vi "7-JUNKOLDOCU.vi"() -> ()   [LabVIEW 2010]
uses:
  7-OCU/7.0-Global.vi
  7-OCU/TabEnum.ctl
  6-OCU Neurons/6.1-UDP Saitek.ctl
  6-OCU Neurons/MDF LatLong.ctl
  6-OCU Neurons/6.1-Act.ctl
  <vilib>/Utility/inputDevices.llb/joystickAcquire.vi
panel:
  in  "Stop Loops 2":bool
  out "Ogrid":u8[][](graph)
  out "MDF Array Out":T1[](array[typedef]) {"Latitude (waypoint)" format="%#_8g"; "Longitude  (waypoint)" format="%#_8g"}
  out "PlanMission":bool
  out "initialized MDF":T1[](array[typedef]) {"Latitude (waypoint)" format="%#_8g"; "Longitude  (waypoint)" format="%#_8g"}
  out "Process loop":bool
  out "AutoMode":bool
  out "ManualMode":bool
  in  "Stop Loops":bool
  out "Startup&Shutdown":bool
  out "Main Tab":string
  in  "Main Tab Interface":T2
  out "Drive Motor Check":bool
  out "Steer Motor Check":bool
  out "LIDAR Motor Check":bool
  out "Vector Nav Check":bool
  in  "Path":path=path "C:/Users/jmccandless/Documents/Olin/S6 - S11/Robotics/Dave Brain 5/Graphics/PNG/olin_o.png"
  out "ignore me 2":bool
  out "ignore me":bool
  out "Way Point Index":i32
  out "Draw??":bool
  in  "Pen Color":u32(colorbox)=15671808
  in  "Select Pen Attributes":T3={"Width"=1, "Style"=enum."Solid"}
  out "Current Waypoint":T1={"Waypoint #"=2.0, "Latitude (waypoint)"=0.0, "Longitude  (waypoint)"=0.0, "Vel (desired)"=0.0, "Dwell Time"=0.0, "Behavior"=enum."OpenFieldTransit", "Expand1"=0.0, "Expand2"=0.0, "Expand3"=0.0} {"Latitude (waypoint)" format="%#_8g"; "Longitude  (waypoint)" format="%#_8g"}
  in  "RobotSpeed_Leg":dbl(slide) min=0.0 max=4.0 step=0.01 scale=0.0..4.0
  in  "Select Your Behavior":T4(ring)
  in  "Exit Planning":bool
  in  "Load From File":bool
  in  "Save to File":bool
  out "MissionDefFile":picture
  out "Saitek Controler 2":T5 {"Right" scale=-32767.0..32767.0; "Left" scale=-32767.0..32767.0; "Yaw" scale=-32767.0..32767.0; "Roll" scale=-32767.0..32767.0; "Pitch" scale=-32767.0..32767.0}
  out "7.7.1 ManualMode Main Controls":T6 {"6.1-Saitek Controller"."Right" scale=-32767.0..32767.0; "6.1-Saitek Controller"."Left" scale=-32767.0..32767.0; "6.1-Saitek Controller"."Yaw" scale=-32767.0..32767.0; "6.1-Saitek Controller"."Roll" scale=-32767.0..32767.0; "6.1-Saitek Controller"."Pitch" scale=-32767.0..32767.0}
  out "Speed":dbl(knob) scale=0.0..10.0
  out "Heading":dbl(knob) scale=-180.0..180.0
  out "Battery":dbl(slide) scale=0.0..24.0
  out "Time":dbl
  in  "Start Mission":bool
  out "AutoMode Dashboard":T7 {"Battery" scale=0.0..24.0; "Heading" scale=-180.0..180.0; "Speed" scale=0.0..10.0}
  out "7.7.1 AutoMode Main Controls":T6 {"6.1-Saitek Controller"."Right" scale=-32767.0..32767.0; "6.1-Saitek Controller"."Left" scale=-32767.0..32767.0; "6.1-Saitek Controller"."Yaw" scale=-32767.0..32767.0; "6.1-Saitek Controller"."Roll" scale=-32767.0..32767.0; "6.1-Saitek Controller"."Pitch" scale=-32767.0..32767.0}
  out "direction info 2":T8
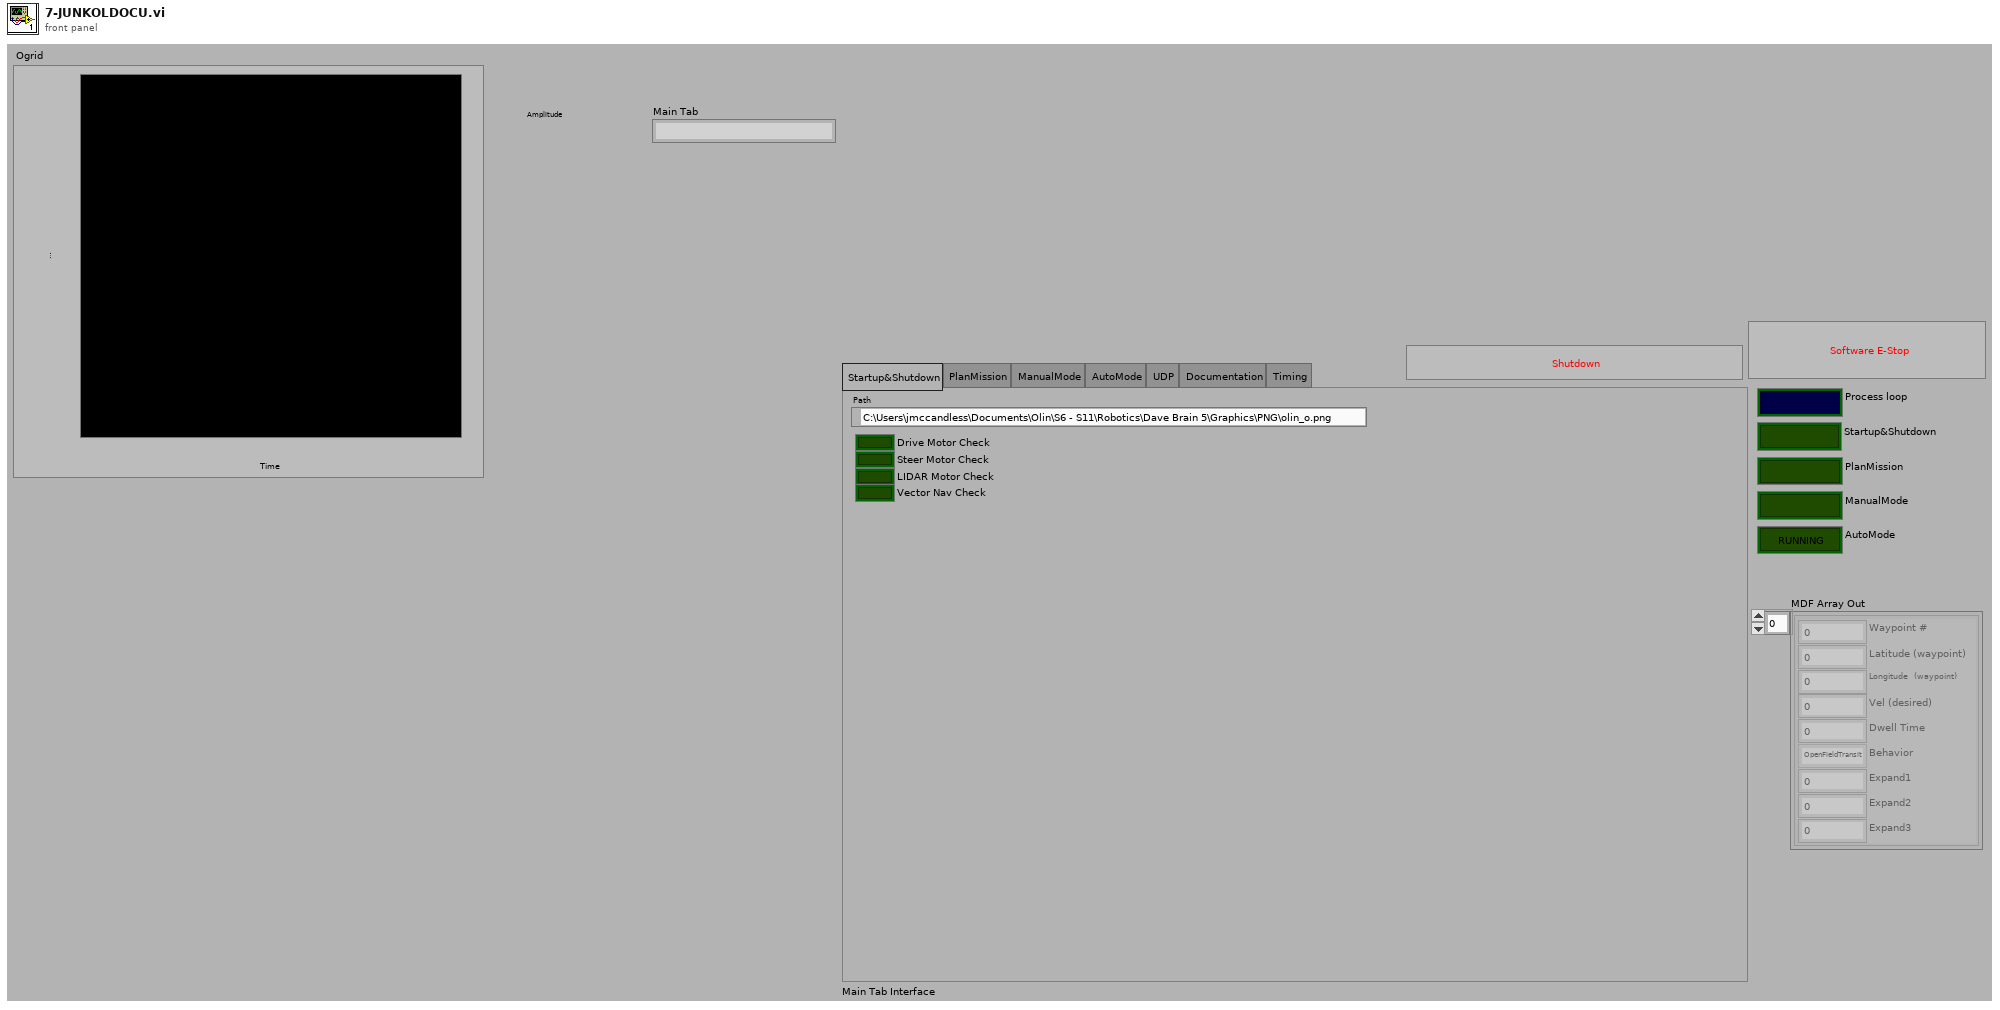
[diagram p1: front panel]
types:
  T1 = typedef "MDF LatLong.ctl" = cluster{"Waypoint #":dbl, "Latitude (waypoint)":ext, "Longitude  (waypoint)":ext, "Vel (desired)":dbl, "Dwell Time":dbl, "Behavior":enum16{"OpenFieldTransit", "WallFollow", "LaneFollow", "ManualMode"}, "Expand1":dbl, "Expand2":dbl, "Expand3":dbl}
  T2 = typedef "TabEnum.ctl" = enum32{"Startup&Shutdown", "PlanMission", "ManualMode", "AutoMode", "UDP", "Documentation", "Timing"}
  T3 = cluster{"Width":u16, "Style":enum32{"Solid", "Dash", "Dot", "DashDot", "DashDotDot"}}
  T4 = enum16{"OpenFieldTransit", "WallFollow", "LaneFollow", "ManualMode"}
  T5 = typedef "6.1-UDP Saitek.ctl" = cluster{"Trig":bool, "2":bool, "3":bool, "4":bool, "5":bool, "6":bool, "7":bool, "8":bool, "9":bool, "10":bool, "11":bool, "Pitch":i32, "Ang":bool[], "Wheel":dbl, "Roll":i32, "Yaw":i32, "Left":i32, "Right":i32}
  T6 = typedef "6.1-Act.ctl" = cluster{"6.1-Saitek Controller":T5, "Joystick Mode":bool, "Shutdown":bool, "Reset":bool, "Begin":bool}
  T7 = cluster{"Speed":dbl, "Heading":dbl, "Battery":dbl, "Time":dbl}
  T8 = cluster{"pov 1":i32, "pov 2":i32, "pov 3":i32, "pov 4":i32}
  T9 = typedef "imagedata.ctl" = cluster{"image type":i32, "image depth":i32, "image":u8[], "mask":u8[], "colors":u32[], "Rectangle":cluster{"left":i16, "top":i16, "right":i16, "bottom":i16}}
  T10 = enum32{"7.1-Act", "7.2-Where", "7.3-What", "7.4-How", "Startup&Shutdown", "PlanMission", "ManualMode", "AutoMode", "UDP", "Documentation", "7.8-Timing"}
  T11 = typedef "LVMouseTypeDef.ctl" = cluster{"Mouse Position":cluster{"X":i32, "Y":i32}, "Mouse Modifiers":cluster{"Button Down":bool, "Shift Mod":bool, "Menu Mod":bool, "Option Mod":bool}}
  T12 = typedef "MDF Array LatLong.ctl" = T1[]
  T13 = cluster{"X axis":i32, "Y axis":i32, "Z axis":i32, "X axis rotation":i32, "Y axis rotation":i32, "Z axis rotation":i32, "U axis":i32, "V axis":i32}
  T14 = cluster{"button 1":bool, "button 2":bool, "button 3":bool, "button 4":bool, "button 5":bool, "button 6":bool, "button 7":bool, "button 8":bool, "button 9":bool, "button 10":bool, "button 11":bool, "button 12":bool, "button 13":bool, "button 14":bool, "button 15":bool, "button 16":bool, "button 17":bool, "button 18":bool, "button 19":bool, "button 20":bool, "button 21":bool, "button 22":bool, "button 23":bool, "button 24":bool, "button 25":bool, "button 26":bool, "button 27":bool, "button 28":bool, "button 29":bool, "button 30":bool, "button 31":bool, "button 32":bool}
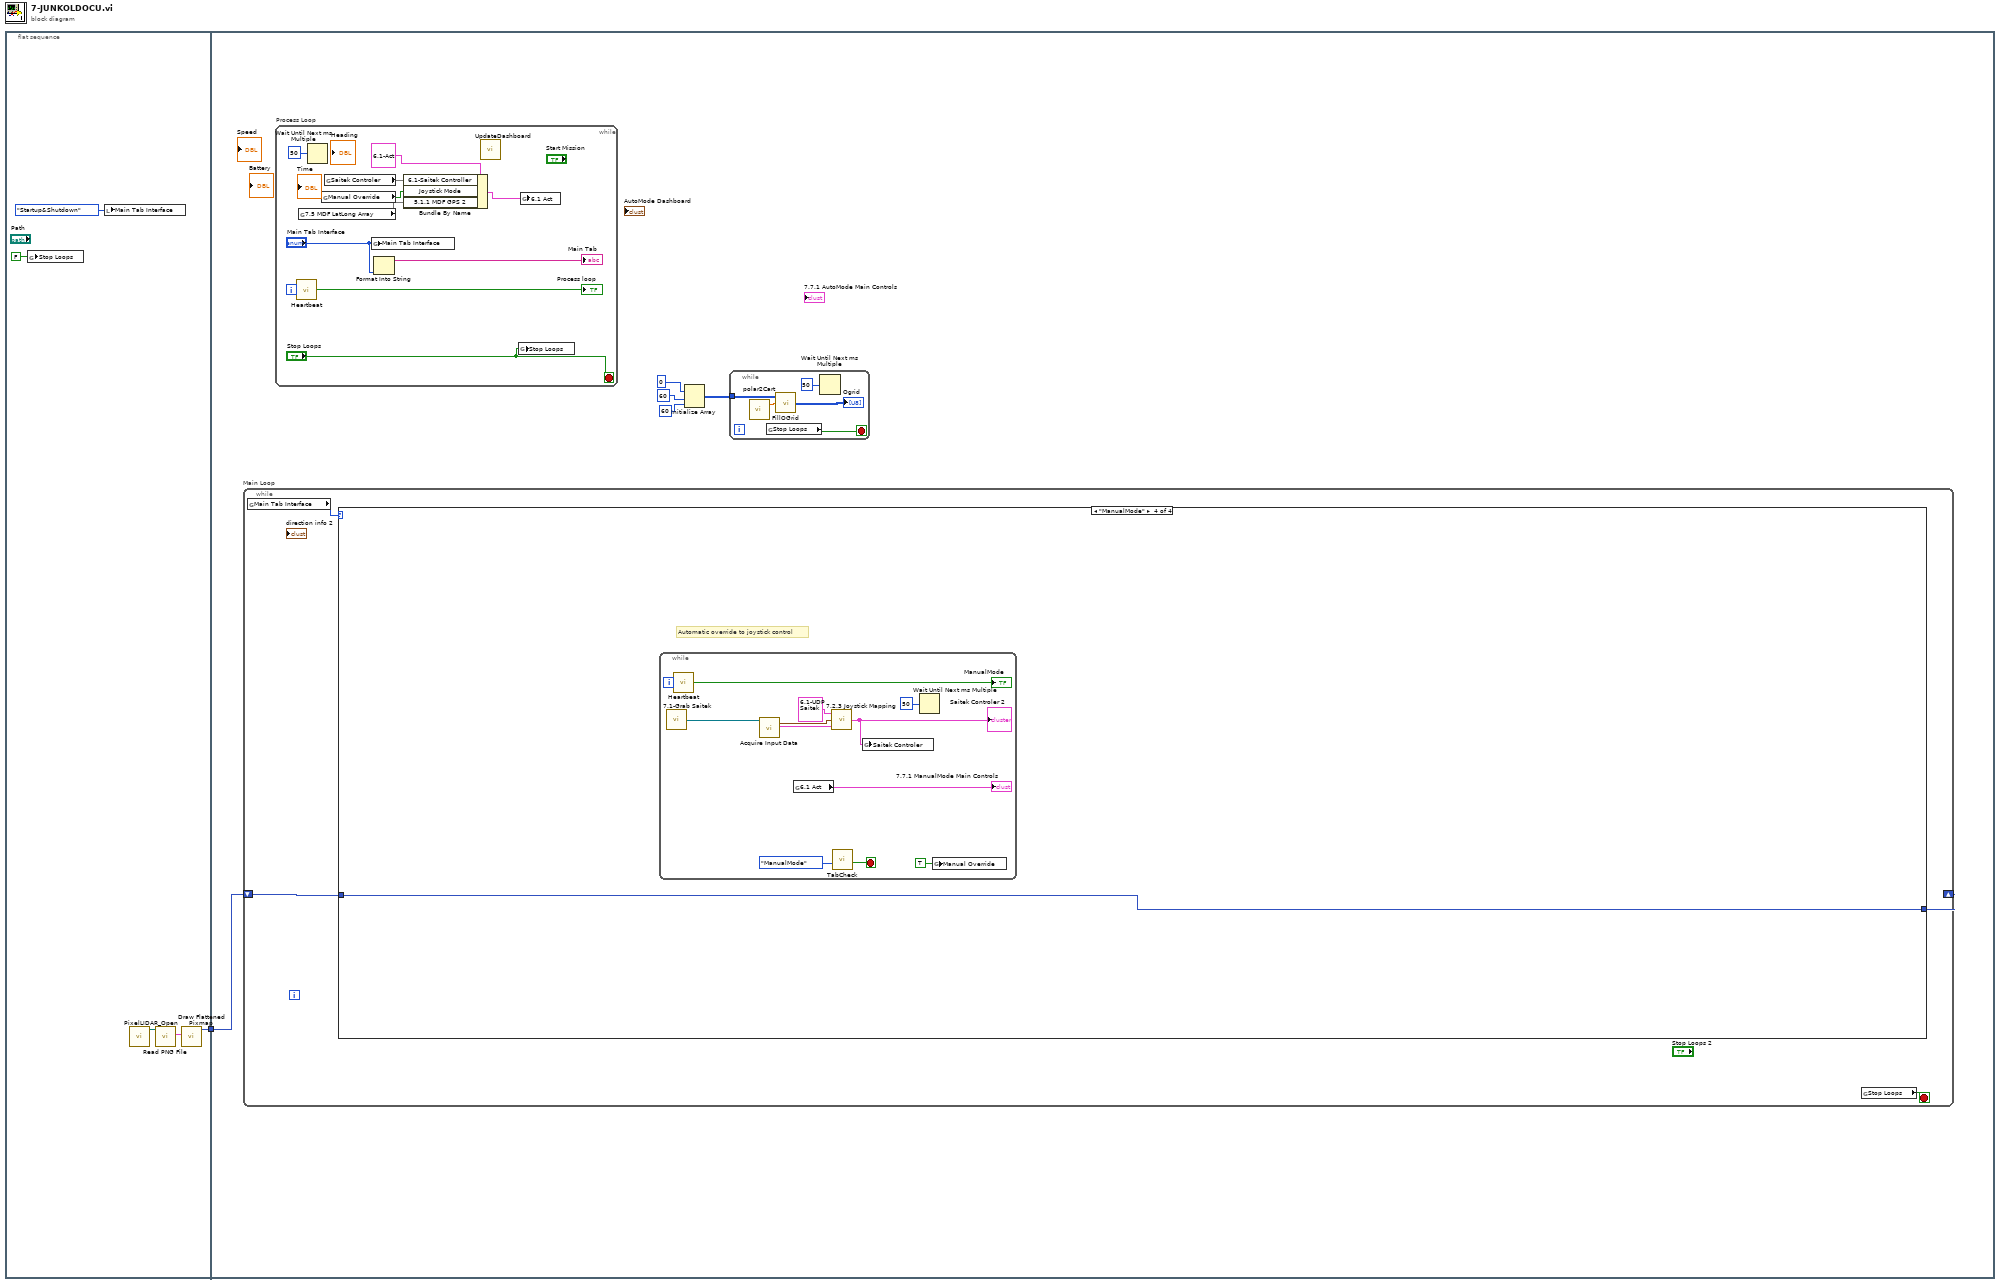
[diagram p0: block diagram]
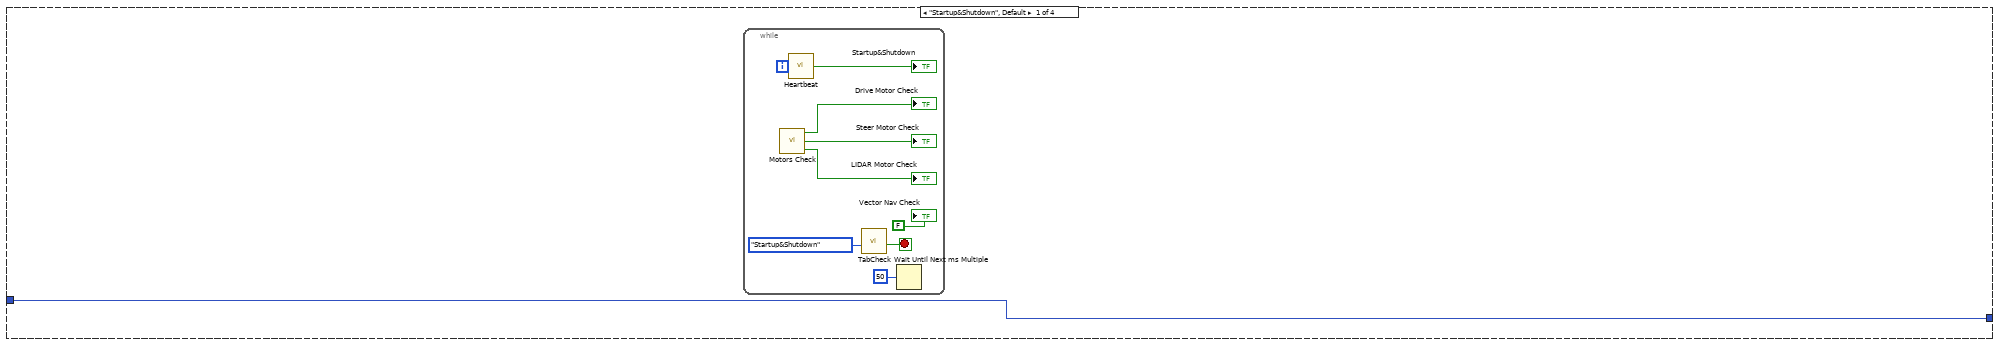
[diagram p2: hidden frame]
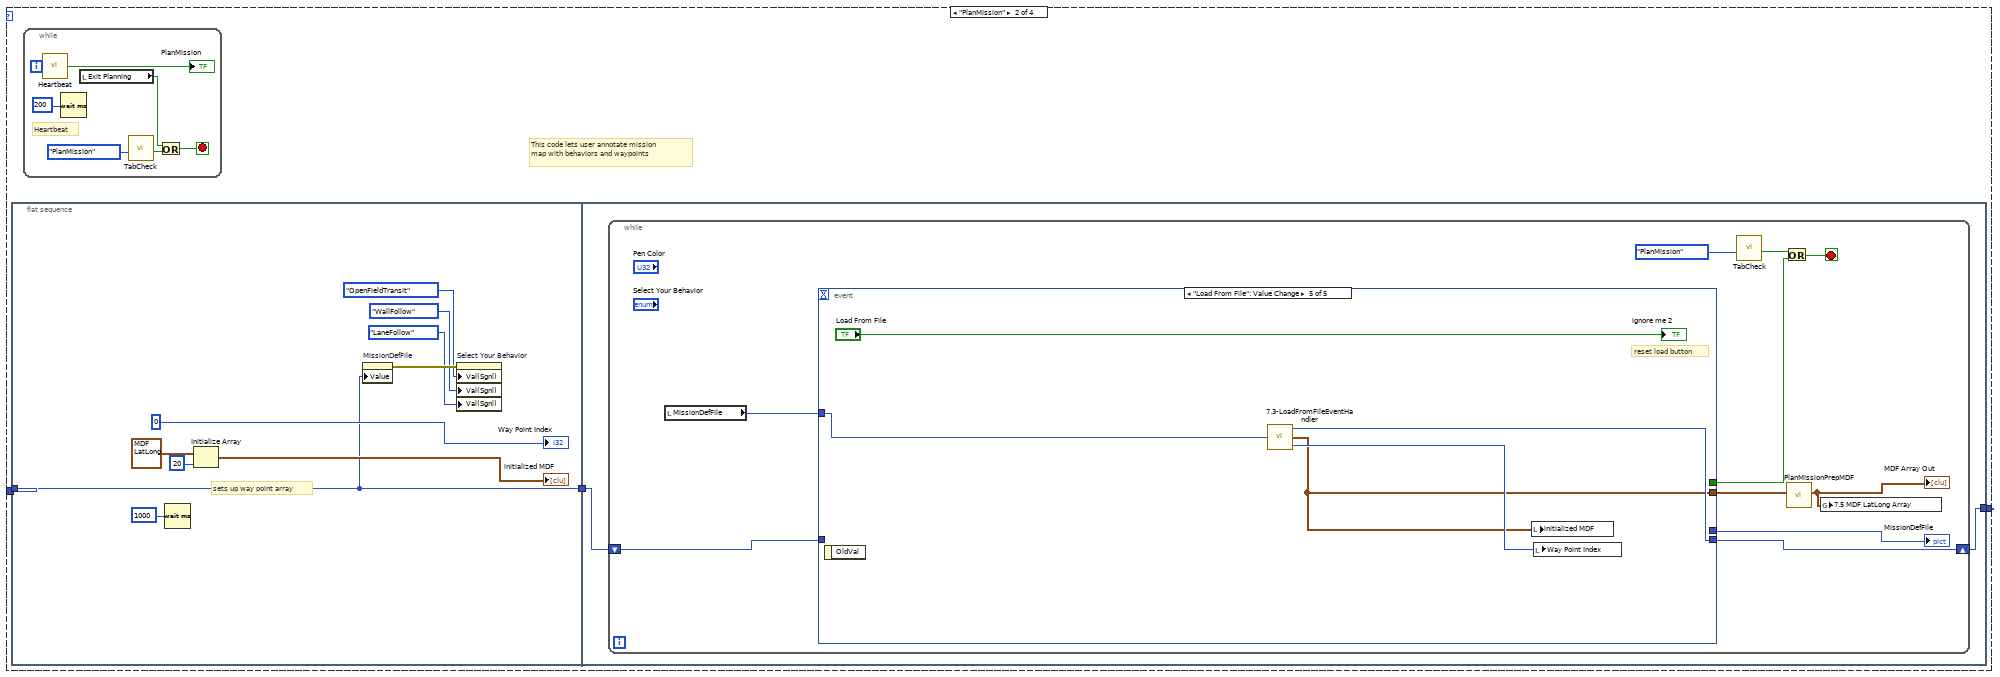
[diagram p3: hidden frame]
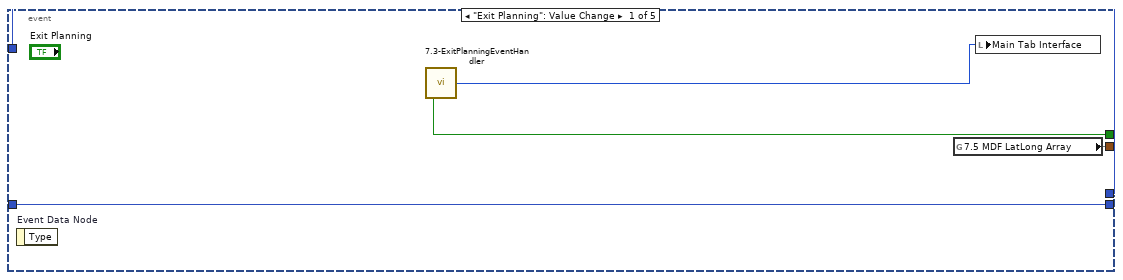
[diagram p4: hidden frame]
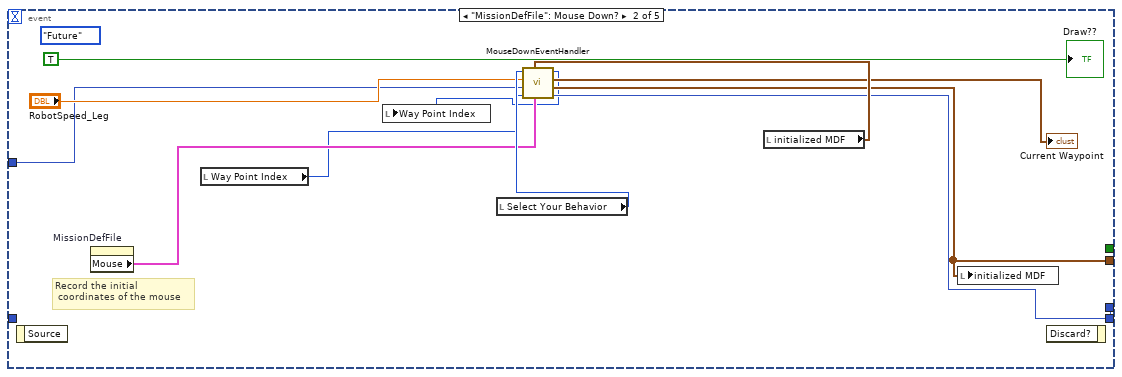
[diagram p5: hidden frame]
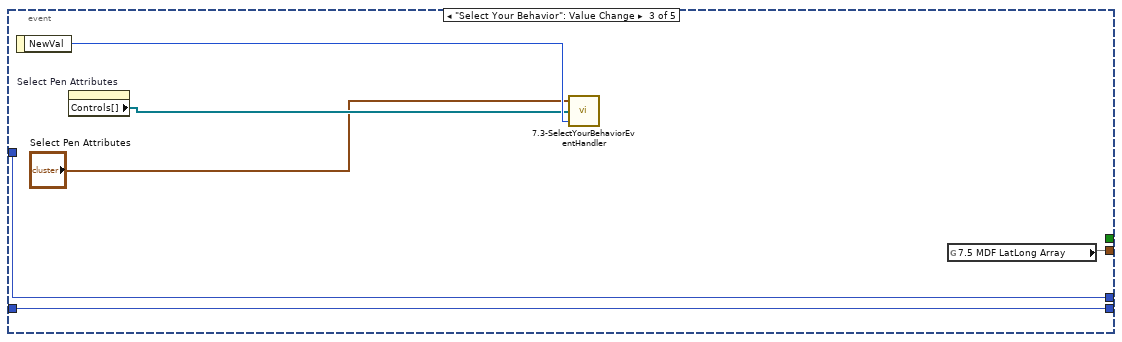
[diagram p6: hidden frame]
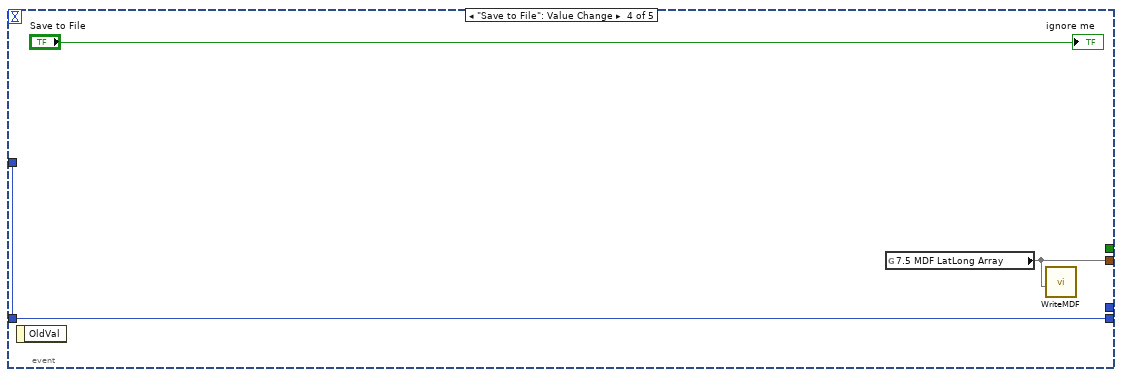
[diagram p7: hidden frame]
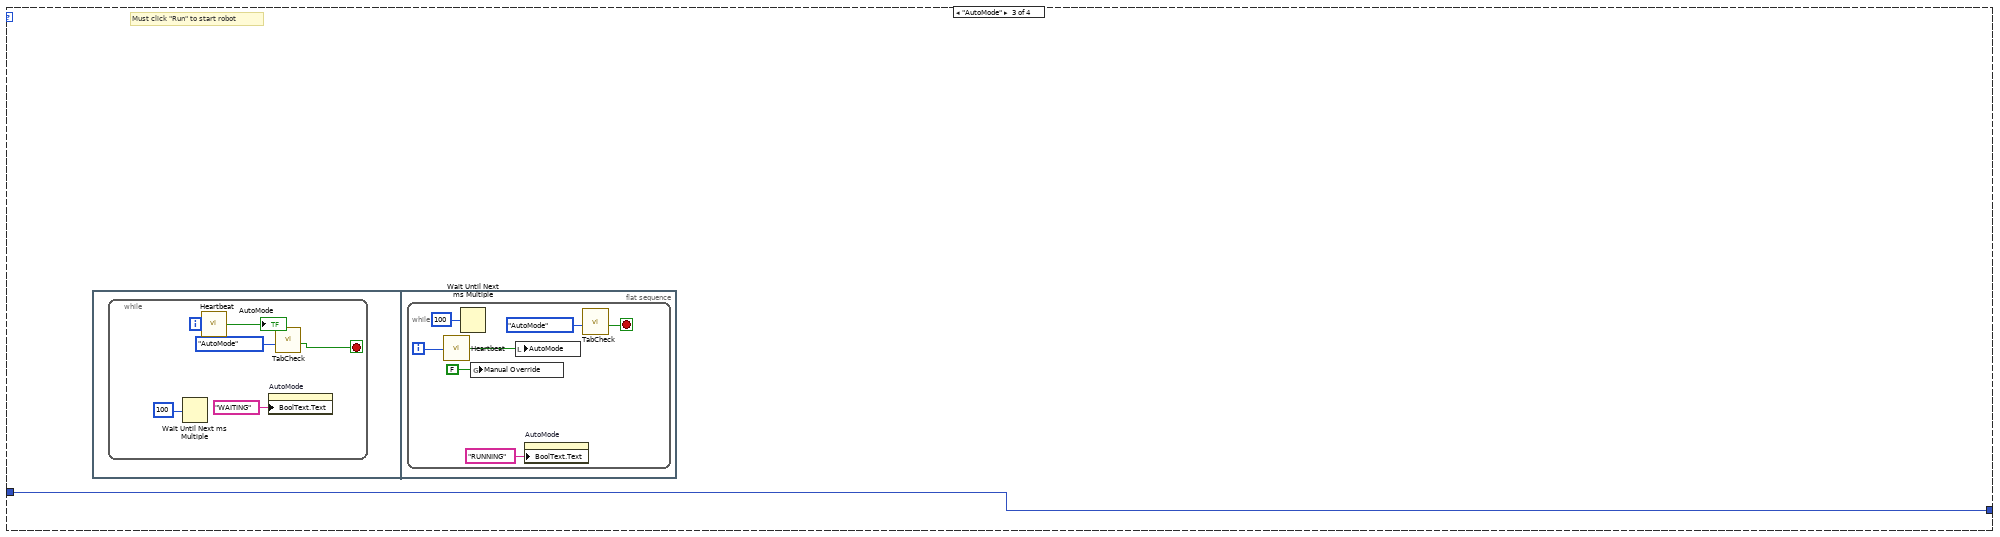
[diagram p8: hidden frame]
diagram:
  n1 = flat-sequence {
    tunnel: [w2] -> w1
    tunnel: w1 -> [w11]
    frame #0 {
      n2 = global write "7.0-Global.vi" "Stop Loops"(FALSE ("Stop Loops")) -> ()
      n3 = local write "Main Tab Interface"(TabEnum."Startup&Shutdown" ("Main Tab Interface  2")) -> ()
      n4 = call "PixelLIDAR_Open.vi"() -> ("MissionMap"=w3:path)  [unwired: 2 in, 3 out]
      n5 = call <vilib>:"Read PNG File.vi"("path to PNG file"=w3) -> ("image data"=w4:T9)  [unwired: 8 in, 2 out]
      n6 = call <vilib>:"Draw Flattened Pixmap.vi"("image data"=w4) -> ("new picture"=w2:picture)  [unwired: 8 in]
    }
    frame #1 {
      n7 = while "Main Loop" {
        shift-right: [w30] -> _
        shift-left: w11 -> [w29]
        stop <- w31 stop-if-true
        n8 = global read "7.0-Global.vi" "Main Tab Interface"() -> (w28:T10)
        n9 = case shown="\"ManualMode\"" w28 {
          tunnel: [w32 w42 w104 w118] -> w30
          tunnel: w29 -> [w32 w44 w104 w118]
          frame "Startup&Shutdown", Default {
            n10 = while {
              i -> [w37]
              stop <- w35 stop-if-true
              n11 = call "Motors Check.vi"() -> ("LIDAR Motor Check"=→"LIDAR Motor Check":bool, "Steer Motor Check"=→"Steer Motor Check":bool, "Drive Motor Check"=→"Drive Motor Check":bool)  [unwired: 4 in]
              n12 = call "Heartbeat.vi"("Loop Iteration"=w37) -> ("Running?"=→"Startup&Shutdown":bool)
              n13 = call "TabCheck.vi"("What I think the tab is"=TabEnum."Startup&Shutdown" ("Main Tab Interface  2")) -> ("Stop current loop"=w35:bool)  [unwired: 9 in]
              n14 = Wait Until Next ms Multiple(millisecond multiple=u32 50) -> ()  [unwired: 1 out]
              "Vector Nav Check" <- FALSE ("Vector Nav Check")
            }
          }
          frame "PlanMission" {
            # "This code lets user annotate mission  map with behaviors and waypoints"
            n15 = flat-sequence {
              tunnel: w44 -> [w46]
              tunnel: [w46] -> w43
              tunnel: w43 -> [w56]
              tunnel: [w55] -> w42
              frame #0 {
                # "sets up way point array"
                n16 = Wait (ms)(milliseconds to wait=u32 1000) -> ()  [unwired: 1 out]
                n17 = Initialize Array ("Initialize WaypointArray")(T1 {"Waypoint #"=0.0, "Latitude (waypoint)"=0.0, "Longitude  (waypoint)"=0.0, "Vel (desired)"=0.0, "Dwell Time"=0.0, "Behavior"=enum."OpenFieldTransit", "Expand1"=0.0, "Expand2"=0.0, "Expand3"=0.0} ("MissionDefinitionFile"), 20 ("dimension size")) -> (→"initialized MDF":T1[])
                n18 = property on="MissionDefFile" class="Pict"("Value"=w46) -> (error out=w50:errorcluster)  [unwired: 2 in, 1 out]
                n19 = property on="Select Your Behavior" class="Enum (strict)"(error in=w50, "Val(Sgnl)"=T4."OpenFieldTransit" ("Select Your Behavior"), "Val(Sgnl)"=T4."WallFollow" ("Value (Signaling)"), "Val(Sgnl)"=T4."LaneFollow" ("Select Your Behavior")) -> ()  [unwired: 1 in, 2 out]
                "Way Point Index" <- 0 ("Boundary Point Index")
              }
              frame #1 {
                n20 = while {
                  shift-right: [w65] -> w55
                  shift-left: w56 -> [w66]
                  stop <- w59 stop-if-true
                  n21 = local read "MissionDefFile"() -> (w64:picture)
                  n22 = event shown="[4] \"Load From File\": Value Change" {
                    selector: _ -> [_ _ _ _ _]
                    dyn-events: _ -> [_ _ _ _ _]
                    timeout: _ -> [_ _ _ _ _]
                    tunnel: [w71 w74 w84 w91 w93] -> w65
                    tunnel: w66 -> [w71 _ w84 _ _]
                    tunnel: [w69 _ _ _ _] -> w60
                    tunnel: [w67 w76 w83 w89 w92] -> w58
                    tunnel: w64 -> [w70 w73 w85 w91 w94]
                    tunnel: [w70 w74 w85 _ _] -> w63
                    event "Exit Planning": Value Change {
                      n23 = event-data "Event Data Node"() -> ()  [unwired: 1 in, 1 out]
                      n24 = call "7.3-ExitPlanningEventHandler.vi"() -> ("Main Tab Interface  2"=w68:T2, "T button?"=w69:bool)
                      n25 = global read "7.0-Global.vi" "7.5 MDF LatLong Array"() -> (w67)
                      n26 = local write "Main Tab Interface"(w68) -> ()
                    }
                    event "MissionDefFile": Mouse Down? {
                      (unwired) enum16{"Past", "Current", "Future"}."Future" ("Status")
                      # "Record the initial\n coordinates of the mouse"
                      n27 = event-data() -> ()  [unwired: 1 in, 1 out]
                      n28 = property on="MissionDefFile" class="Pict"() -> ("Mouse"=w80:T11)  [unwired: 2 in, 2 out]
                      n29 = local read "Way Point Index"() -> (w78:i32)
                      n30 = local read "Select Your Behavior"() -> (w81:T4)
                      n31 = local read "initialized MDF"() -> (w77:T1[])
                      n32 = call "MouseDownEventHandler.vi"("Mouse"=w80, "initialized MDF 2"=w77, "Way Point Index"=w78, "MissionDefFile"=w73, "RobotSpeed_Leg"="RobotSpeed_Leg", "Behavior"=w81) -> ("new picture"=w74:picture, "initialized MDF"=w76:T1[], "MDFile"=→"Current Waypoint":T1, "Numeric"=w72:i32)
                      n33 = local write "Way Point Index"(w72) -> ()
                      n34 = local write "initialized MDF"(w76) -> ()
                      n35 = event-data() -> ()  [unwired: 2 in, 1 out]
                      "Draw??" <- TRUE ("Draw??")
                    }
                    event "Select Your Behavior": Value Change {
                      n36 = event-data() -> ("NewVal"=w88:T4)  [unwired: 1 in]
                      n37 = property on="Select Pen Attributes" class="Clust (strict)"() -> ("Controls[]"=w87:refnum<vi>[])  [unwired: 2 in, 2 out]
                      n38 = call "7.3-SelectYourBehaviorEventHandler.vi"("NewVal"=w88, "Controls[]"=w87, "Select Pen Attributes"="Select Pen Attributes") -> ()
                      n39 = global read "7.0-Global.vi" "7.5 MDF LatLong Array"() -> (w83)
                    }
                    event "Save to File": Value Change {
                      n40 = event-data() -> ()  [unwired: 1 in, 1 out]
                      n41 = global read "7.0-Global.vi" "7.5 MDF LatLong Array"() -> (w89)
                      n42 = call "WriteMDF.vi"("MDF In"=w89) -> ()  [unwired: 11 in]
                      "ignore me" <- "Save to File"
                    }
                    event "Load From File": Value Change {
                      # "reset load button"
                      n43 = event-data() -> ()  [unwired: 1 in, 1 out]
                      n44 = call "7.3-LoadFromFileEventHandler.vi"("MissionDefFile"=w94) -> ("Number of Waypoints Read"=w95:i32, "MDF Out"=w92:T12, "new picture"=w93:picture)
                      n45 = local write "initialized MDF"(w92) -> ()
                      n46 = local write "Way Point Index"(w95) -> ()
                      "ignore me 2" <- "Load From File"
                    }
                  }
                  "MissionDefFile" <- w63
                  n47 = call "TabCheck.vi"("What I think the tab is"=TabEnum."PlanMission" ("Main Tab Interface  2")) -> ("Stop current loop"=w61:bool)  [unwired: 9 in]
                  n48 = Or(x=w61, y=w60) -> (x .or. y?=w59:bool)
                  n49 = call "PlanMissionPrepMDF.vi"("MDF Array In"=w58) -> ("MDF Array Out"=w57:T1[])  [unwired: 10 in]
                  "MDF Array Out" <- w57
                  n50 = global write "7.0-Global.vi" "7.5 MDF LatLong Array"(w57) -> ()
                }
              }
            }
            n51 = while {
              i -> [w101]
              stop <- w97 stop-if-true
              # "Heartbeat"
              n52 = call "Heartbeat.vi"("Loop Iteration"=w101) -> ("Running?"=→"PlanMission":bool)
              n53 = Wait (ms)(milliseconds to wait=u32 200) -> ()  [unwired: 1 out]
              n54 = local read "Exit Planning"() -> (w98:bool)
              n55 = call "TabCheck.vi"("What I think the tab is"=TabEnum."PlanMission" ("Main Tab Interface  2")) -> ("Stop current loop"=w99:bool)  [unwired: 9 in]
              n56 = Or(x=w98, y=w99) -> (x .or. y?=w97:bool)
            }
          }
          frame "AutoMode" {
            # "Must click \"Run\" to start robot"
            n57 = flat-sequence {
              frame #0 {
                n58 = while {
                  i -> [w107]
                  stop <- w105 stop-if-true
                  n59 = Wait Until Next ms Multiple(millisecond multiple=u32 100) -> ()  [unwired: 1 out]
                  n60 = call "Heartbeat.vi"("Loop Iteration"=w107) -> ("Running?"=→"AutoMode":bool)
                  n61 = property on="AutoMode" class="Bool (strict)"("BoolText.Text"="WAITING" ("Boolean Text.Text")) -> ()  [unwired: 2 in, 2 out]
                  n62 = call "TabCheck.vi"("What I think the tab is"=TabEnum."AutoMode" ("Main Tab Interface  2")) -> ("Stop current loop"=w105:bool)  [unwired: 9 in]
                }
              }
              frame #1 {
                n63 = while {
                  i -> [w115]
                  stop <- w112 stop-if-true
                  n64 = call "Heartbeat.vi"("Loop Iteration"=w115) -> ("Running?"=w114:bool)
                  n65 = Wait Until Next ms Multiple(millisecond multiple=u32 100) -> ()  [unwired: 1 out]
                  n66 = global write "7.0-Global.vi" "Manual Override"(FALSE ("Manual Override")) -> ()
                  n67 = local write "AutoMode"(w114) -> ()
                  n68 = property on="AutoMode" class="Bool (strict)"("BoolText.Text"="RUNNING" ("Boolean Text.Text")) -> ()  [unwired: 2 in, 2 out]
                  n69 = call "TabCheck.vi"("What I think the tab is"=TabEnum."AutoMode" ("Main Tab Interface  2")) -> ("Stop current loop"=w112:bool)  [unwired: 9 in]
                }
              }
            }
          }
          frame "ManualMode" {
            # "Automatic override to joystick control"
            n70 = while {
              i -> [w129]
              stop <- w127 stop-if-true
              n71 = call "7.1-Grab Saitek.vi"() -> ("Saitek ID"=w121:refnum<k1>)
              n72 = call "Heartbeat.vi"("Loop Iteration"=w129) -> ("Running?"=→"ManualMode":bool)
              n73 = call-poly <vilib>:"Acquire Input Data.vi"("device ID"=w121) -> ("axis info"=w123:T13, "button info"=w124:T14)  [unwired: 14 in, 3 out]
              n74 = global read "7.0-Global.vi" "6.1 Act"() -> (→"7.7.1 ManualMode Main Controls":T6)
              n75 = call "7.2.3 Joystick Mapping.vi"("button info"=w124, "axis info"=w123, 3:T5 {"Trig"=FALSE, "2"=FALSE, "3"=FALSE, "4"=FALSE, "5"=FALSE, "6"=FALSE, "7"=FALSE, "8"=FALSE, "9"=FALSE, "10"=FALSE, "11"=FALSE, "Pitch"=0, "Ang"=[], "Wheel"=0.0, "Roll"=0, "Yaw"=0, "Left"=0, "Right"=0} ("Saitek Controler 2")) -> ("Joystick Out"=w120:T5)
              "Saitek Controler 2" <- w120
              n76 = call "TabCheck.vi"("What I think the tab is"=TabEnum."ManualMode" ("Main Tab Interface  2")) -> ("Stop current loop"=w127:bool)  [unwired: 9 in]
              n77 = global write "7.0-Global.vi" "Saitek Controler"(w120) -> ()
              n78 = Wait Until Next ms Multiple(millisecond multiple=u32 50) -> ()  [unwired: 1 out]
              n79 = global write "7.0-Global.vi" "Manual Override"(TRUE ("Manual Override")) -> ()
            }
          }
        }
        n80 = global read "7.0-Global.vi" "Stop Loops"() -> (w31:bool)
      }
      n81 = while "Process Loop" {
        i -> [w23]
        stop <- "Stop Loops" stop-if-true
        n82 = call "Heartbeat.vi"("Loop Iteration"=w23) -> ("Running?"=→"Process loop":bool)
        n83 = global read "7.0-Global.vi" "7.5 MDF LatLong Array"() -> (w18)
        n84 = Wait Until Next ms Multiple(millisecond multiple=u32 50) -> ()  [unwired: 1 out]
        n85 = global read "7.0-Global.vi" "Manual Override"() -> (w19:bool)
        n86 = global read "7.0-Global.vi" "Saitek Controler"() -> (w20)
        n87 = global write "7.0-Global.vi" "Main Tab Interface"("Main Tab Interface") -> ()
        n88 = Format Into String("Main Tab Interface") -> (resulting string=→"Main Tab":string)  [unwired: 3 in, 1 out]
        n89 = Bundle By Name(cluster=T6 {"6.1-Saitek Controller"={"Trig"=FALSE, "2"=FALSE, "3"=FALSE, "4"=FALSE, "5"=FALSE, "6"=FALSE, "7"=FALSE, "8"=FALSE, "9"=FALSE, "10"=FALSE, "11"=FALSE, "Pitch"=0, "Ang"=[], "Wheel"=0.0, "Roll"=0, "Yaw"=0, "Left"=0, "Right"=0}, "Joystick Mode"=FALSE, "Shutdown"=FALSE, "Reset"=FALSE, "Begin"=FALSE} ("Main Controls"), "6.1-Saitek Controller"=w20, "Joystick Mode"=w19, "5.1.1 MDF GPS 2"=w18) -> (w17:T6)
        n90 = call "UpdateDashboard.vi"() -> ()  [unwired: 12 in]
        n91 = global write "7.0-Global.vi" "Stop Loops"("Stop Loops") -> ()
        n92 = global write "7.0-Global.vi" "6.1 Act"(w17) -> ()
      }
      n93 = Initialize Array(u8 0 ("element"), 60 ("dimension size"), 60 ("dimension size")) -> (w10:u8[][])
      n94 = while {
        tunnel: w10 -> [w14]
        stop <- w13 stop-if-true
        n95 = call "polar2Cart.vi"() -> ("X"=w16:dbl[])  [unwired: 1 in, 1 out]
        n96 = global read "7.0-Global.vi" "Stop Loops"() -> (w13:bool)
        n97 = call "FillOGrid.vi"("X"=w16, "OGrid In"=w14) -> ("OGrid Out"=→"Ogrid":u8[][])  [unwired: 1 in]
        n98 = Wait Until Next ms Multiple(millisecond multiple=u32 50) -> ()  [unwired: 1 out]
      }
    }
  }
